vi "picoGetTimebase.vi"(6 "Memory Segment":u32, 8 "error in (no error)":errorcluster, 10 "Rapid Block Acquisition Settings":T1={"preTriggerSamples"=0, "postTriggerSamples"=90000, "timebase"=1, "Down-Sample Mode"=4, "Down Sample Ratio"=90, "Oversample"=1, "Number of Captures"=250} {"Down Sample Ratio" min=1 step=1; "Down-Sample Mode" items=["None"=0, "Aggregate"=1, "Decimate"=2, "Average"=4]}, 11 "handle in":i16) -> (0 "error out":errorcluster, 1 "Sample Interval":sgl, 3 "handle out":i16)   [LabVIEW 2011]
uses:
  PS2000a.dll
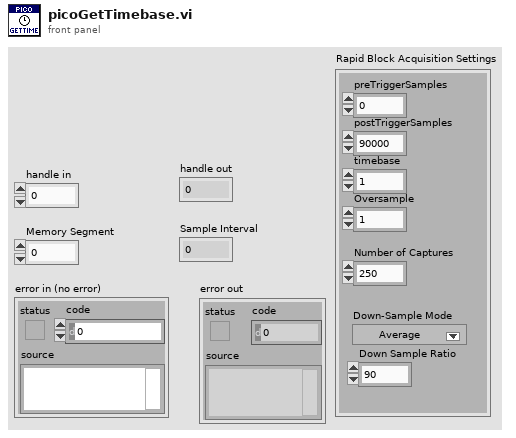
[diagram p1: front panel]
types:
  T1 = cluster{"preTriggerSamples":u32, "postTriggerSamples":u32, "timebase":u32, "Down-Sample Mode":i32, "Down Sample Ratio":u32, "Oversample":i16, "Number of Captures":u32}
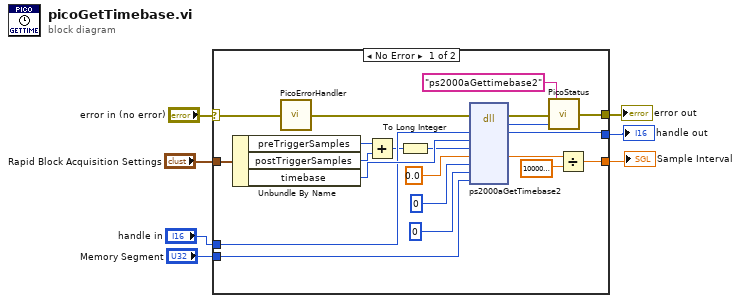
[diagram p0: block diagram]
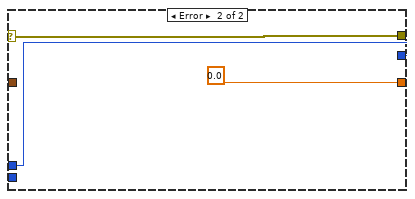
[diagram p2: hidden frame]
diagram:
  n1 = case shown="No Error" "error in (no error)" {
    selector: "error in (no error)" -> [w19 w31]
    tunnel: [w18 w31] -> w3
    tunnel: [w17 w30] -> w4
    tunnel: "Memory Segment" -> [w11 _]
    tunnel: "handle in" -> [w16 w30]
    tunnel: "Rapid Block Acquisition Settings" -> [w10 _]
    tunnel: [w8 sgl 0.0] -> w1
    frame No Error {
      n2 = Unbundle By Name(w10) -> ("preTriggerSamples"=w22:u32, "postTriggerSamples"=w23:u32, "timebase"=w24:u32)
      n3 = call "PicoErrorHandler.vi"("error in"=w19) -> ("error out"=w26:errorcluster)
      n4 = Add(x=w22, y=w23) -> (x+y=w12:u32)
      n5 = To Long Integer(number=w12) -> (32bit integer=w9:i32)
      n6 = dll-call lib="ps2000a.dll" fn="ps2000aGetTimebase2"(error in=w26, "handle"=w16, "timebase"=w24, "noSamples"=w9, "timeIntervalNanoseconds"=sgl 0.0, "oversample"=i16 0, "maxSamples"=0, "segmentIndex"=w11) -> (error out=w25:errorcluster, "PICO_STATUS"=w20:u32, "handle"=w17:i16, "timeIntervalNanoseconds"=w27:sgl)  [unwired: 7 in, 1 out]
      n7 = call "PicoStatus.vi"("PICO STATUS"=w20, "error in"=w25, "source"="ps2000aGettimebase2") -> ("error out"=w18:errorcluster)
      n8 = Divide(x=w27, y=sgl 1000000000.0) -> (x/y=w8:sgl)
    }
    frame Error {
    }
  }
  "error out" <- w3
  "handle out" <- w4
  "Sample Interval" <- w1
